vi "Control Servo.vi"(8 "error in (no error)":errorcluster, 9 "setpoint (V)":dbl, 10 "force (V)":dbl, 11 "Simulated Controller in":refnum<class "Simulated Controller.lvclass">) -> (0 "error out":errorcluster, 2 "servo pw (us)":dbl, 3 "Simulated Controller out":refnum<class "Simulated Controller.lvclass">)   [LabVIEW 2020, in "Simulated Controller.lvclass"]
uses:
  Simulated Controller.lvclass
  <vilib>/numeric/Random Number (Range) DBL.vi
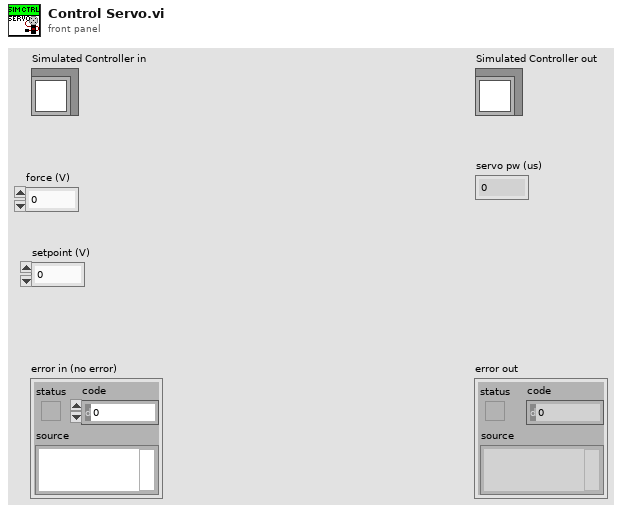
[diagram p1: front panel]
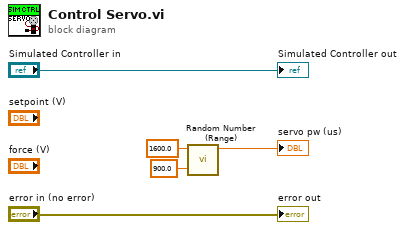
[diagram p0: block diagram]
diagram:
  n1 = call-poly <vilib>:"Random Number (Range).vi"("lower bound (0)"=900.0, "upper bound (100)"=1600.0) -> ("number"=→"servo pw (us)":dbl)  [unwired: 9 in]
  "error out" <- "error in (no error)"
  "Simulated Controller out" <- "Simulated Controller in"
